vi "Process_data.vi"(4 "Measurement top level?":bool) -> (6 "Vel stat display":string[][](table), 7 "First Plot data Cluster":cluster{"X array":dbl[], "Y array":dbl[]}[](array[cluster]), 8 "Second Plot Data Cluster":cluster{"X array":dbl[], "Y array":dbl[]}[](array[cluster]), 9 "Max Measurement time up":bool)   [LabVIEW 2017]
uses:
  Controls/Instrument_Array.ctl
  Controls/Inst_type.ctl
  Controls/Post_Process.ctl
  Controls/User_Specific_mode.ctl
  Controls/Server_Comms.ctl
  Globals/Meas_global.vi
  Globals/LDA_meas_global_1.vi
  Globals/Dynamic_call_global.ph.vi
  Acquisition/PWA/PWAtasksGLOBAL.vi
  Globals/Trav_pos_global.vi
  Globals/Preference_global.vi
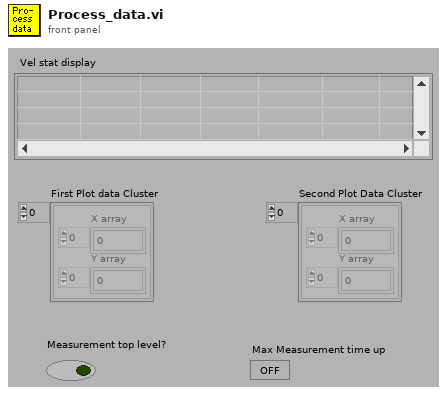
[diagram p1: front panel]
types:
  T1 = typedef "LDA_Setup.ctl" = cluster{"dimensions":enum16{"1D", "2D"}, "Analogue Freq Multiplier":dbl}
  T2 = typedef "PWA_Data.ctl" = enum16{"No PWA Data", "One Ch PWA"}
  T3 = typedef "Instrument_Array.ctl" = enum16{"PWA", "LDA", "Analogue"}
  T4 = typedef "Inst_type.ctl" = enum16{"Propeller anemometer", "Raw voltage", "Pressure Transducer", "Pitot-static tube", "Preston tube", "Hot wire", "Cross wire 1", "Cross wire 2", "Generic Linear", "Generic Polynomial", "Generic BackPoly", "Fast FID", "Thermocouple", "Cold wire", "Pulsed Wire", "LDA Vel", "LDA Tran time", "LDA Arr time", "Microphone"}
  T5 = typedef "Post_Process.ctl" = enum16{"Take New Data", "Post Process Raw Data File"}
  T6 = typedef "User_Specific_mode.ctl" = enum16{"Check VI only", "Run VI"}
  T7 = enum16{"Save no data", "Save data in new files", "Save data in existing files"}
  T8 = typedef "Server_Comms.ctl" = enum16{"Server Link Healthy", "Do Not Link To Server"}
  T9 = typedef "Trigger_Mode.ctl" = enum16{"Free Running", "Start on Trigger", "Trigger Every Block", "Trigger Every Sample"}
  T10 = typedef "Analysis_info_cluster.ctl" = cluster{"Colour":u32, "Inst type":T4, "Inst name":string, "Symbol":string, "Code name":string, "Extra Info":string, "Inst Array":T3, "Extra Titles":string[], "Extra Values":string[], "U":dbl, "u^2":dbl, "u^3":dbl, "u^4":dbl, "Skew_u":dbl, "Kurt_u":dbl, "Sd Error in Mean":dbl, "% u'/U":dbl, "X":dbl, "Y":dbl, "Z":dbl, "Timescale integral Estimate":dbl, "Sd Error in Variance":dbl, "Calib File":path, "Calib Constants":dbl[], "Output Position":bool, "Full Stats":bool, "Av Sampling Rate":dbl, "Av No of Samples":dbl, "Total Meas Time (s)":dbl, "ADAM Ch Name":string, "Max value":dbl, "Min value":dbl}
  T11 = typedef "Time_Trace_Cluster.ctl" = cluster{"Weighting":dbl[], "Time (s)":dbl[], "Voltage":dbl[], "Eng Values":dbl[]}
  T12 = typedef "Shift_Cluster.ctl" = cluster{"Stats":dbl[], "Spectra_Auto":dbl[], "Histogram":dbl[], "Hist Max":dbl, "Hist Min":dbl, "No of Samples":i32, "No in plume":i32, "Weight sum":dbl, "No Of Hist bins":i32, "TimeTrace Max":dbl, "Time Trace Min":dbl, "Trace St Deviation":dbl}
  T13 = typedef "Cross_Moments_Shift_Cluster.ctl" = cluster{"Stats":dbl[], "Resampled No of Samples":i32, "Resampled delta T":dbl, "Cross Correlation":dbl[]}
  T14 = typedef "Correlation_cluster1.ctl" = cluster{"U inst":string, "uw":dbl, "u^2w":dbl, "uw^2":dbl, "uw/u'w'":dbl, "W inst":string, "uw^3":dbl, "u^3w":dbl, "u^2w^2":dbl, "Index U":i32, "Index W":i32, "Error info":string[]}
  T15 = typedef "Traverse_cluster.ctl" = cluster{"Start X":sgl, "Start Y":sgl, "Start Z":sgl, "End X":sgl, "End Y":sgl, "End Z":sgl, "No. of pts.":i32, "Spacing":T16, "Filename":path, "Tunnel Speed":dbl, "Averaging time (min)":dbl, "Extra Commands":string, "Carrier_1 Q (l/min)":dbl, "Carrier_2 Q (l/min)":dbl, "Trace Gas Concentration (%)":dbl, "Specific Arguments":string, "Comments":string, "Row No":i32, "Row Type Selector":T17, "Completion time":string, "Row Duration (mins)":dbl, "No. of Valid pts.":i32, "Meas Setup File":string}
  T16 = typedef "Spacing.ctl" = enum16{"Linear", "Log", "Gauss", "Specified", "N/A"}
  T17 = typedef "Multi_run_mode.ctl" = enum16{"Move Traverse Only", "Set Tunnel Speed Only", "Set Source Only", "Set Measurement Conditions", "Single Measurement", "Vertical Profile", "Lateral Profile", "Longitudinal Profile", "Explore Volume", "Multi-Axis Profile", "Auto Calibrate", "Meas Fast FID Bkgnd", "Check Beam Power", "Scanning Valve Measurement", "Run VI Named:", "Set ADAM Ch", "Wait (minutes)", "Send Message", "Synchronize With:", "Fall Back to this Row", "Turn Off Row Repeating", "Blank Row", "Traverse 3D Volume"}
  T18 = typedef "Graph_Type.ctl" = enum16{"Show no graph", "Voltage trace", "Velocity trace", "Vel histogram", "Spectrum", "f.E(f) v Log f", "Auto-Corr"}
  T19 = cluster{"Plot 1":u16, "Plot 2":u16, "Save graph":u16, "Plot Type":T18}
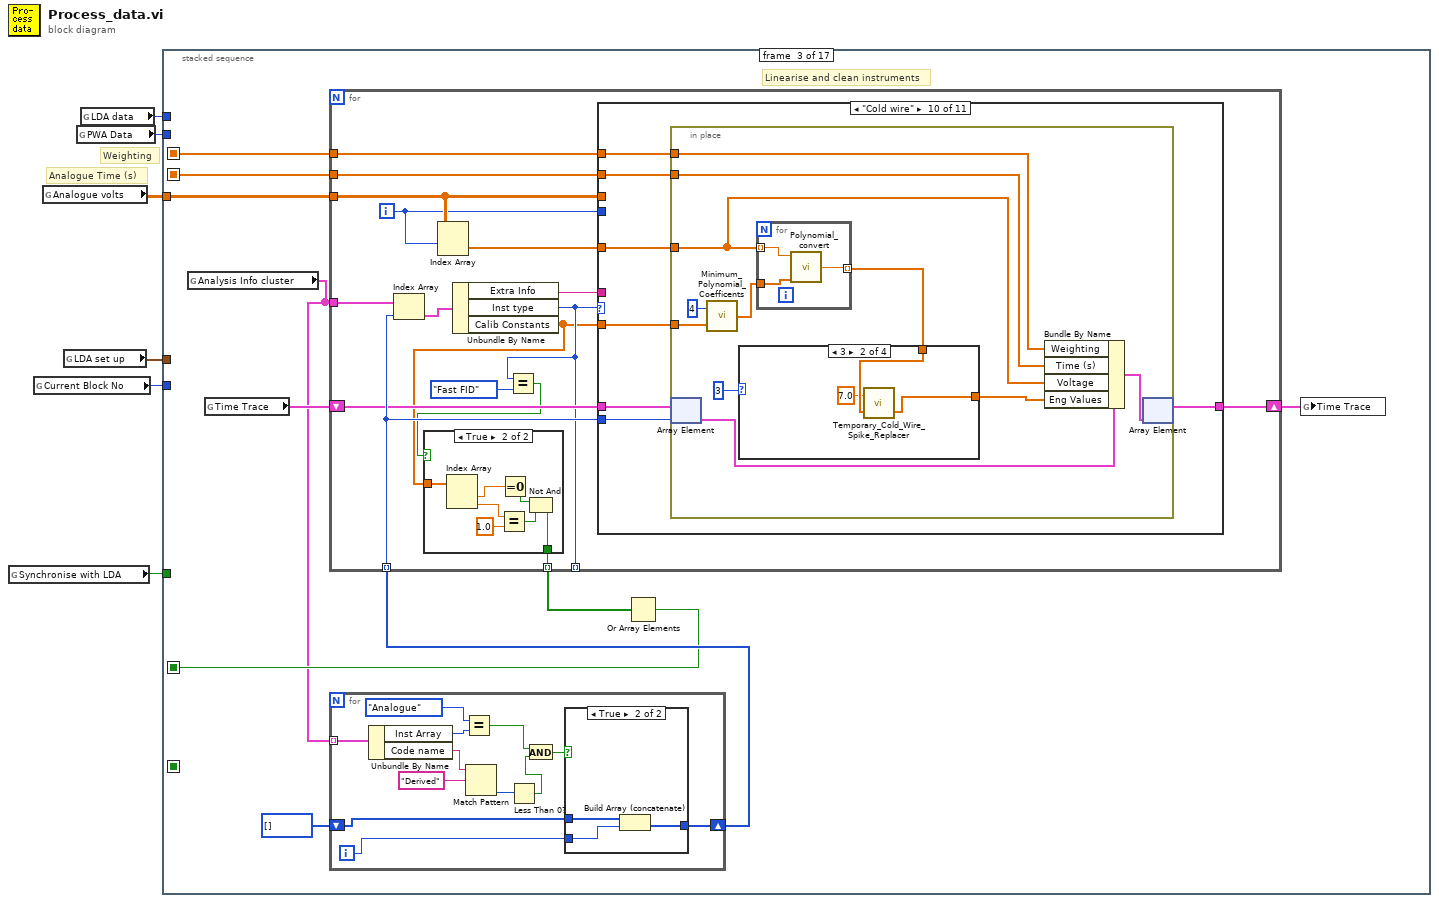
[diagram p0: block diagram]
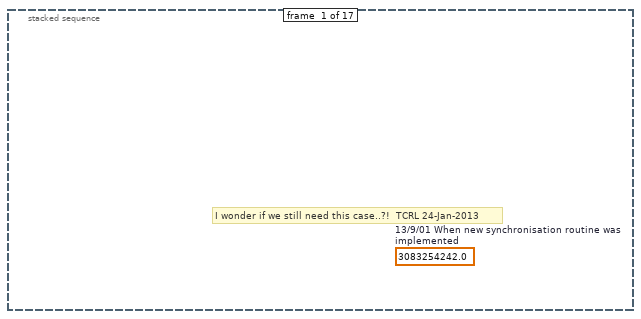
[diagram p2: hidden frame]
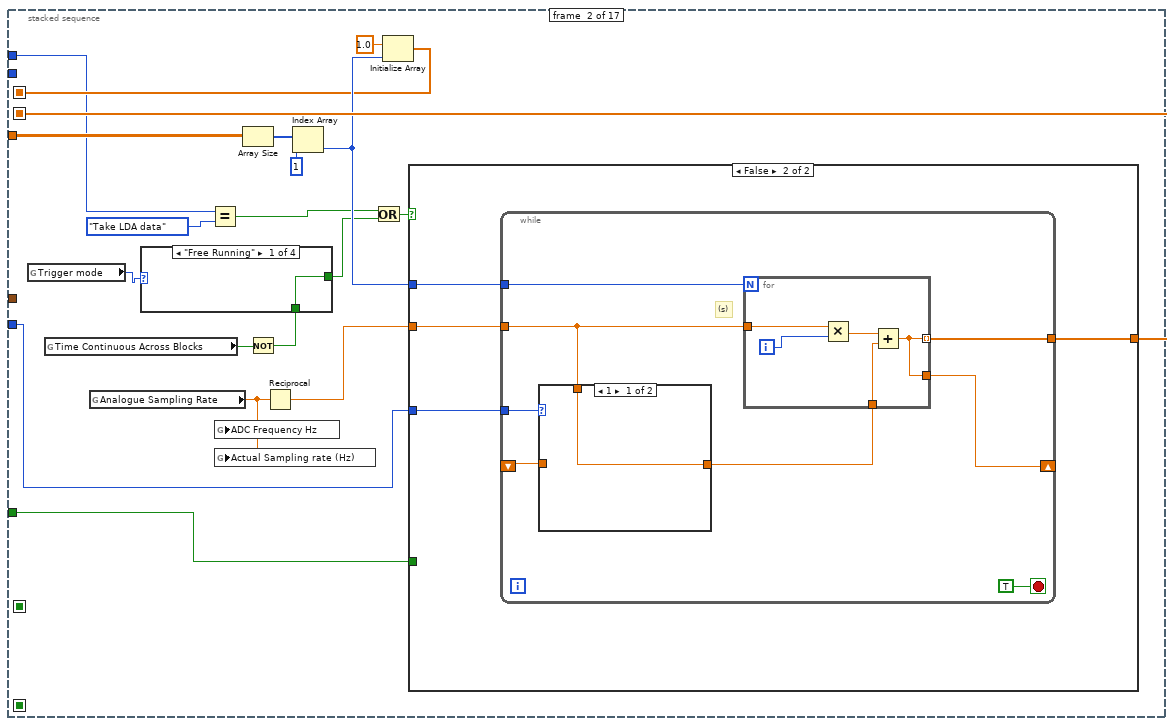
[diagram p3: hidden frame]
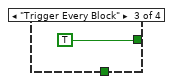
[diagram p5: hidden frame]
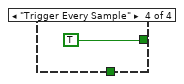
[diagram p6: hidden frame]
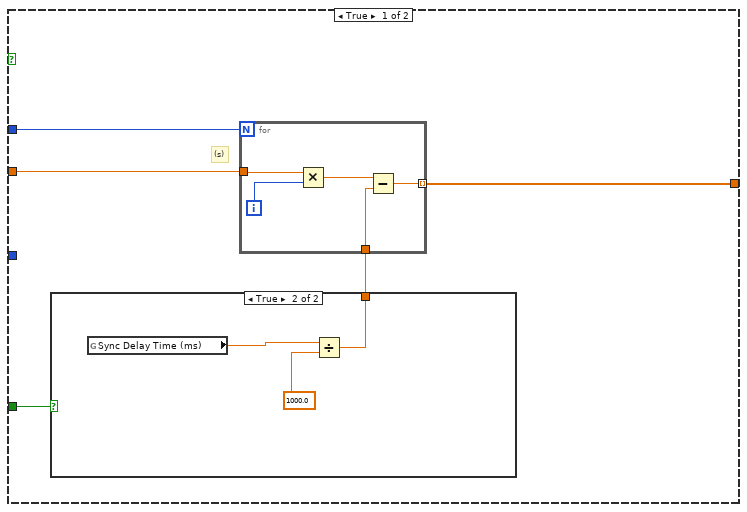
[diagram p7: hidden frame]
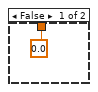
[diagram p8: hidden frame]
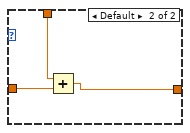
[diagram p9: hidden frame]
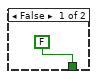
[diagram p11: hidden frame]
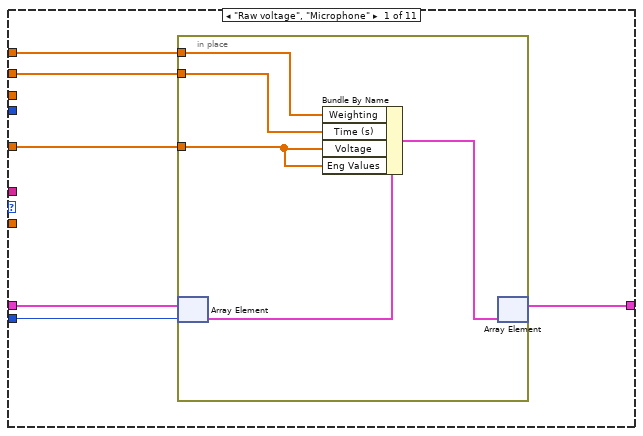
[diagram p12: hidden frame]
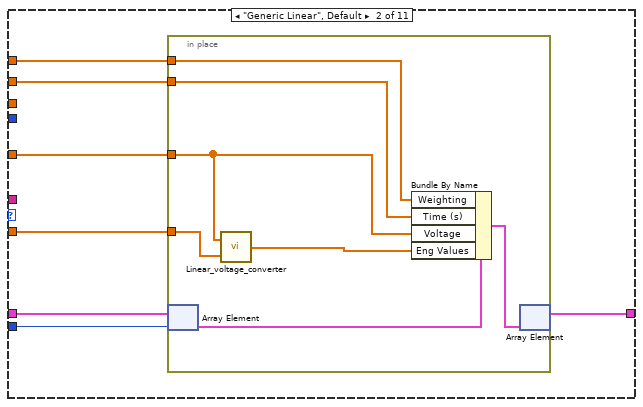
[diagram p13: hidden frame]
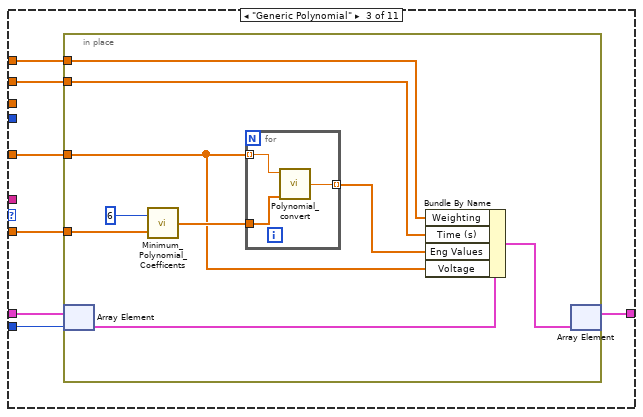
[diagram p14: hidden frame]
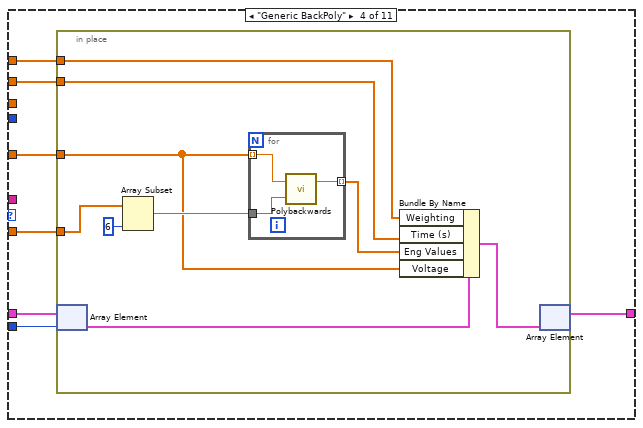
[diagram p15: hidden frame]
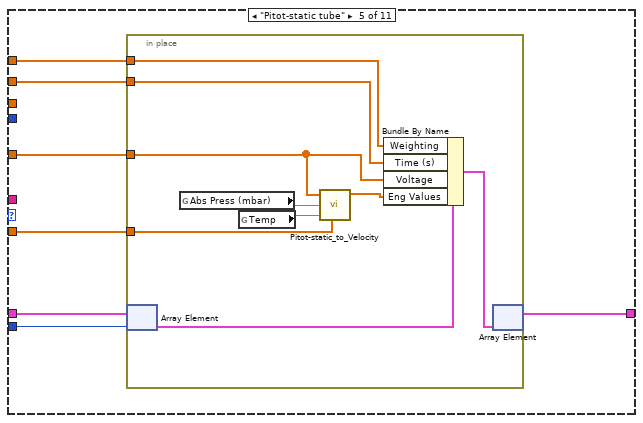
[diagram p16: hidden frame]
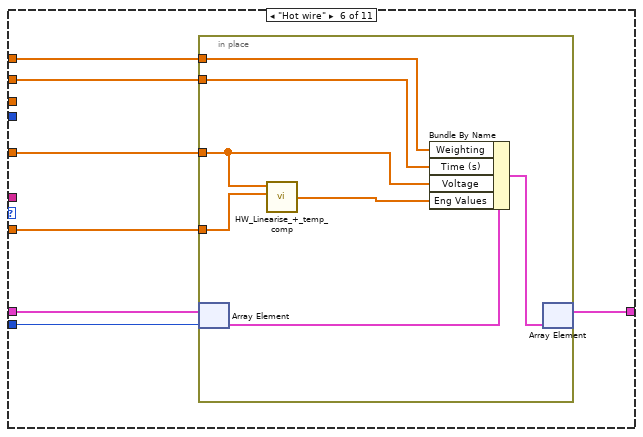
[diagram p17: hidden frame]
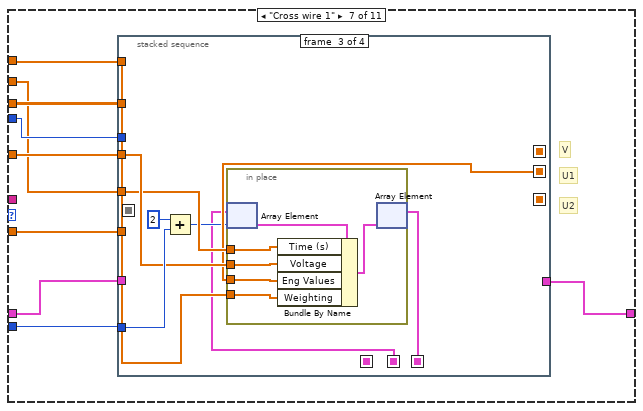
[diagram p18: hidden frame]
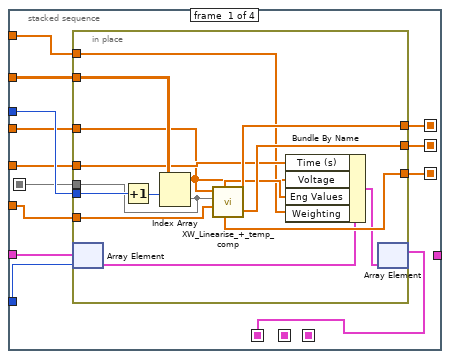
[diagram p19: hidden frame]
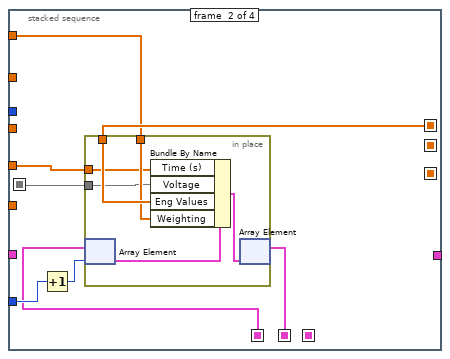
[diagram p20: hidden frame]
diagram:
  # "Weighting"
  # "Analogue Time (s)"
  n1 = global read "Meas_global.vi" "Synchronise with LDA"() -> (w4:bool)
  n2 = global read "Meas_global.vi" "Current Block No"() -> (w5:i32)
  n3 = global read "Meas_global.vi" "Analogue volts"() -> (w2:dbl[][])
  n4 = global read "Meas_global.vi" "LDA set up"() -> (w1:T1)
  n5 = global read "Meas_global.vi" "PWA Data"() -> (w3:T2)
  n6 = global read "Meas_global.vi" "LDA data"() -> (w6:enum16{"No LDA data", "Take LDA data"})
  n7 = stacked-sequence {
    seq-local: [_ w22 _ _ _ _ _ _ _ _ _ _ _ _ _ _ _] -> [_ _ w71 _ _ _ _ _ _ _ _ _ _ _ _ _ _]
    seq-local: [_ w19 _ _ _ _ _ _ _ _ _ _ _ _ _ _ _] -> [_ _ w70 _ _ _ _ _ _ _ _ _ _ _ _ _ _]
    seq-local: [_ _ w67 _ _ _ _ _ _ _ _ _ _ _ _ _ _] -> [_ _ _ _ _ w441 _ _ _ _ _ _ _ _ _ _ _]
    seq-local: [_ _ _ _ _ _ _ _ _ _ _ _ _ _ _ w709 _] -> [_ _ _ _ _ _ _ _ _ _ _ _ _ _ _ _ w735]
    tunnel: w5 -> [_ w15 _ _ _ _ w445 _ _ _ _ _ _ _ _ _ _]
    tunnel: w6 -> [_ w12 _ w383 _ _ _ _ _ _ _ _ _ _ _ w710 _]
    tunnel: w2 -> [_ w25 w74 _ _ _ _ _ _ _ _ _ w660 _ _ _ _]
    tunnel: w4 -> [_ w16 _ w382 _ _ _ _ _ _ _ _ _ _ _ _ _]
    tunnel: w3 -> [_ _ _ _ _ _ w448 _ _ _ _ _ _ _ _ _ _]
    tunnel: w1 -> [_ _ _ w380 _ _ _ _ _ _ _ _ _ _ _ _ _]
    frame #0 {
      (unwired) 3083254242.0  # 13/9/01 When new synchronisation routine was implemented
      # "I wonder if we still need this case..?!  TCRL 24-Jan-2013"
    }
    frame #1 {
      n8 = global read "Meas_global.vi" "Trigger mode"() -> (w14:T9)
      n9 = global read "Meas_global.vi" "Time Continuous Across Blocks"() -> (w8:bool)
      n10 = global read "Meas_global.vi" "Analogue Sampling Rate"() -> (w18:dbl)
      n11 = Equal?(x=w12, y=enum16{"No LDA data", "Take LDA data"}."Take LDA data" ("LDA data")) -> (x = y?=w10:bool)
      n12 = global write "LDA_meas_global_1.vi" "ADC Frequency Hz"(w18) -> ()
      n13 = global write "Meas_global.vi" "Actual Sampling rate (Hz)"(w18) -> ()
      n14 = Array Size(array=w25) -> (size(s)=w24:i32[])
      n15 = Not(x=w8) -> (.not. x?=w7:bool)
      n16 = case shown="\"Free Running\"" w14 {
        tunnel: [w26 w27 TRUE TRUE] -> w9
        tunnel: w7 -> [w26 w27 _ _]
        frame "Free Running" {
        }
        frame "Start on Trigger" {
        }
        frame "Trigger Every Block" {
        }
        frame "Trigger Every Sample" {
        }
      }
      n17 = Reciprocal(x=w18) -> (1/x=w17:dbl)
      n18 = Index Array(array=w24, index=1) -> (element=w21:i32)
      n19 = Or(x=w10, y=w9) -> (x .or. y?=w11:bool)
      n20 = Initialize Array(1.0 ("element"), w21) -> (w19:dbl[])
      n21 = case shown="False" w11 {
        tunnel: [w34 w47] -> w22
        tunnel: w21 -> [w33 w46]
        tunnel: w17 -> [w31 w45]
        tunnel: w16 -> [w30 _]
        tunnel: w15 -> [_ w44]
        frame True {
          # "(s)"
          n22 = case shown="True" w30 {
            tunnel: [0.0 w37] -> w32
            frame False {
            }
            frame True {
              n23 = global read "LDA_meas_global_1.vi" "Sync Delay Time (ms)"() -> (w38:dbl)
              n24 = Divide(x=w38, y=1000.0) -> (x/y=w37:dbl)
            }
          }
          n25 = for {
            N: w33 -> [_]
            tunnel: w31 -> [w42]
            tunnel: [w41] -> w34 mode=indexing
            tunnel: w32 -> [w39]
            i -> [w43]
            n26 = Multiply(x=w42, y=w43) -> (x*y=w40:dbl)
            n27 = Subtract(x=w40, y=w39) -> (x-y=w41:dbl)
          }
        }
        frame False {
          n28 = while {
            tunnel: [w55] -> w47
            tunnel: w46 -> [w54]
            tunnel: w45 -> [w48]
            tunnel: w44 -> [w52]
            shift-right: [w50] -> _
            shift-left: _ -> [w49]
            stop <- TRUE stop-if-true
            # "(s)"
            n29 = case shown="1" w52 {
              tunnel: [w56 w57] -> w51
              tunnel: w49 -> [_ w59]
              tunnel: w48 -> [w56 w58]
              frame 1 {
              }
              frame Default {
                n30 = Add(x=w58, y=w59) -> (x+y=w57:dbl)
              }
            }
            n31 = for {
              N: w54 -> [_]
              tunnel: w48 -> [w64]
              tunnel: [w61] -> w55 mode=indexing
              tunnel: w51 -> [w62]
              tunnel: [w61] -> w50
              i -> [w60]
              n32 = Multiply(x=w64, y=w60) -> (x*y=w63:dbl)
              n33 = Add(x=w63, y=w62) -> (x+y=w61:dbl)
            }
          }
        }
      }
    }
    frame #2 {
      # "Linearise and clean instruments"
      n34 = global read "Meas_global.vi" "Analysis Info cluster"() -> (w66:T10[])
      n35 = global read "Meas_global.vi" "Time Trace"() -> (w69:T11[])
      n36 = for {
        tunnel: w66 -> [w78] mode=indexing
        shift-right: [w75] -> w72
        shift-left: i32[] [] -> [w76]
        i -> [w77]
        n37 = Unbundle By Name(w78) -> ("Inst Array"=w86:T3, "Code name"=w84:string)
        n38 = Equal?(x=Instrument_Array."Analogue" ("Inst Array"), y=w86) -> (x = y?=w80:bool)
        n39 = Match Pattern(string=w84, regular expression="Derived") -> (offset past match=w82:i32)  [unwired: 4 out]
        n40 = Less Than 0?(x=w82) -> (x < 0?=w81:bool)
        n41 = And(x=w80, y=w81) -> (x .and. y?=w79:bool)
        n42 = case shown="True" w79 {
          tunnel: w77 -> [_ w90]
          tunnel: w76 -> [w87 w89]
          tunnel: [w87 w88] -> w75
          frame False {
          }
          frame True {
            n43 = Build Array (concatenate)(w89, w90) -> (w88:i32[])
          }
        }
      }
      n44 = for {
        tunnel: w74 -> [w106]
        tunnel: [w94] -> _ mode=indexing
        tunnel: w72 -> [w102] mode=indexing
        shift-right: [w98] -> w68
        shift-left: w69 -> [w101]
        tunnel: w71 -> [w99]
        tunnel: w70 -> [w105]
        tunnel: w66 -> [w104]
        tunnel: [w91] -> w65 mode=indexing
        i -> [w97]
        n45 = Index Array(array=w104, index=w102) -> (element=w103:T10)
        n46 = Index Array(array=w106, index (row)=w97) -> (element=w100:dbl[])  [unwired: 1 in]
        n47 = Unbundle By Name(w103) -> ("Extra Info"=w96:string, "Inst type"=w94:T4, "Calib Constants"=w93:dbl[])
        n48 = Equal?(x=w94, y=Inst_type."Fast FID" ("Inst type")) -> (x = y?=w92:bool)
        n49 = case shown="True" w92 {
          tunnel: w93 -> [_ w114]
          tunnel: [FALSE w108] -> w91
          frame False {
          }
          frame True {
            n50 = Index Array(array=w114) -> (element #1=w113:dbl, element #2=w112:dbl)  [unwired: 2 in]
            n51 = Equal?(x=w112, y=1.0) -> (x = y?=w110:bool)
            n52 = Equal To 0?(x=w113) -> (x = 0?=w109:bool)
            n53 = Not And(1:w110, 2:w109) -> (0:w108:bool)
          }
        }
        n54 = case shown="\"Cold wire\"" w94 {
          tunnel: w93 -> [_ w132 w145 w165 w184 w200 w215 _ w295 w326 w363]
          tunnel: w97 -> [_ _ _ _ _ _ w216 _ _ _ _]
          tunnel: w106 -> [_ _ _ _ _ _ w213 _ _ _ _]
          tunnel: w99 -> [w115 w126 w144 w161 w178 w194 w210 _ w290 w322 w357]
          tunnel: w100 -> [w116 w131 w146 w164 w183 w199 w214 _ w294 w327 w362]
          tunnel: w102 -> [w119 w130 w142 w162 w180 w195 w212 _ w292 w321 w359]
          tunnel: w101 -> [w120 w128 w141 w163 w181 w197 w211 w288 w293 w325 w360]
          tunnel: [w117 w127 w140 w159 w179 w196 w209 w288 w291 w324 w358] -> w98
          tunnel: w105 -> [w118 w129 w143 w160 w182 w198 w208 _ w289 w323 w361]
          tunnel: w96 -> [_ _ _ _ _ _ _ _ _ _ w356]
          frame "Raw voltage", "Microphone" {
            n55 = in-place {
              in-place-border: w118 -> [w121]
              in-place-border: w116 -> [w123]
              in-place-border: w115 -> [w122]
              n56 = in-place-array #1(w120, w119) -> (w124:T11)
              n57 = Bundle By Name(cluster=w124, "Weighting"=w121, "Time (s)"=w122, "Voltage"=w123, "Eng Values"=w123) -> (w125:T11)
              n58 = in-place-array #1(w125) -> (w117:T11[])  [unwired: 1 out]
            }
          }
          frame "Generic Linear", Default {
            n59 = in-place {
              in-place-border: w132 -> [w139]
              in-place-border: w131 -> [w134]
              in-place-border: w129 -> [w133]
              in-place-border: w126 -> [w135]
              n60 = in-place-array #2(w128, w130) -> (w136:T11)
              n61 = call "Linear_voltage_converter.vi"("Caib const A,B"=w139, "Voltage array"=w134) -> ("Converted array"=w138:dbl[])
              n62 = Bundle By Name(cluster=w136, "Weighting"=w133, "Time (s)"=w135, "Voltage"=w134, "Eng Values"=w138) -> (w137:T11)
              n63 = in-place-array #2(w137) -> (w127:T11[])  [unwired: 1 out]
            }
          }
          frame "Generic Polynomial" {
            n64 = in-place {
              in-place-border: w146 -> [w151]
              in-place-border: w145 -> [w154]
              in-place-border: w144 -> [w148]
              in-place-border: w143 -> [w147]
              n65 = in-place-array #3(w141, w142) -> (w150:T11)
              n66 = call "Minimum_Polynomial_Coefficents.vi"("Calib consts"=w154, "Max Length"=6) -> ("Coefficients"=w153:dbl[])
              n67 = for {
                tunnel: w153 -> [w158]
                tunnel: w151 -> [w157] mode=indexing
                tunnel: [w156] -> w152 mode=indexing
                n68 = call "Polynomial_convert.vi"("Calib constants"=w158, "Voltage"=w157) -> ("Eng Values"=w156:dbl)  [unwired: 4 out]
              }
              n69 = Bundle By Name(cluster=w150, "Weighting"=w147, "Time (s)"=w148, "Eng Values"=w152, "Voltage"=w151) -> (w149:T11)
              n70 = in-place-array #3(w149) -> (w140:T11[])  [unwired: 1 out]
            }
          }
          frame "Generic BackPoly" {
            n71 = in-place {
              in-place-border: w165 -> [w174]
              in-place-border: w164 -> [w169]
              in-place-border: w161 -> [w167]
              in-place-border: w160 -> [w166]
              n72 = in-place-array #4(w163, w162) -> (w171:T11)
              n73 = Array Subset(array=w174, length=6) -> (w173:dbl[])  [unwired: 1 in]
              n74 = for {
                tunnel: w173 -> [w177]
                tunnel: w169 -> [w176] mode=indexing
                tunnel: [w175] -> w170 mode=indexing
                n75 = call "Polybackwards.vi"("Coefficients"=w177, "Y input"=w176) -> ("X output"=w175:dbl)  [unwired: 1 out]
              }
              n76 = Bundle By Name(cluster=w171, "Weighting"=w166, "Time (s)"=w167, "Eng Values"=w170, "Voltage"=w169) -> (w168:T11)
              n77 = in-place-array #4(w168) -> (w159:T11[])  [unwired: 1 out]
            }
          }
          frame "Pitot-static tube" {
            n78 = in-place {
              in-place-border: w184 -> [w193]
              in-place-border: w183 -> [w187]
              in-place-border: w182 -> [w185]
              in-place-border: w178 -> [w188]
              n79 = in-place-array #5(w181, w180) -> (w190:T11)
              n80 = global read "Meas_global.vi" "Abs Press (mbar)"() -> (w192:dbl)
              n81 = global read "Meas_global.vi" "Temp"() -> (w186:dbl)
              n82 = call "Pitot-static_to_Velocity.vi"("Pressure Trans voltage"=w187, "Atmos Press mbar  (1000)"=w192, "Temp  C  (20)"=w186, "Pressure Trans Calib const"=w193) -> ("Velocity (m/s)"=w191:dbl[])  [unwired: 1 in, 3 out]
              n83 = Bundle By Name(cluster=w190, "Weighting"=w185, "Time (s)"=w188, "Voltage"=w187, "Eng Values"=w191) -> (w189:T11)
              n84 = in-place-array #5(w189) -> (w179:T11[])  [unwired: 1 out]
            }
          }
          frame "Hot wire" {
            n85 = in-place {
              in-place-border: w200 -> [w207]
              in-place-border: w199 -> [w202]
              in-place-border: w198 -> [w201]
              in-place-border: w194 -> [w203]
              n86 = in-place-array #6(w197, w195) -> (w205:T11)
              n87 = call "HW_Linearise_+_temp_comp.vi"("Caib const"=w207, "HW voltage"=w202) -> ("Velocity"=w206:dbl[])  [unwired: 3 in, 1 out]
              n88 = Bundle By Name(cluster=w205, "Weighting"=w201, "Time (s)"=w203, "Voltage"=w202, "Eng Values"=w206) -> (w204:T11)
              n89 = in-place-array #6(w204) -> (w196:T11[])  [unwired: 1 out]
            }
          }
          frame "Cross wire 1" {
            # "U2"
            # "U1"
            # "V"
            n90 = stacked-sequence {
              seq-local: [w225 _ _ _] -> [_ w250 _ _]
              seq-local: [w224 _ _ _] -> [_ _ w262 _]
              seq-local: [w223 _ _ _] -> [_ _ _ w278]
              seq-local: [_ w245 _ _] -> [_ _ w259 _]
              seq-local: [_ _ w258 _] -> [_ _ _ w274]
              seq-local: [w222 _ _ _] -> [_ w248 _ w277]
              seq-local: [w219 _ _ _] -> [_ w244 _ _]
              tunnel: w216 -> [w229 _ _ _]
              tunnel: w215 -> [w228 _ _ _]
              tunnel: w214 -> [w227 _ w265 _]
              tunnel: w213 -> [w226 _ _ _]
              tunnel: w212 -> [w220 w251 w266 w281]
              tunnel: w211 -> [w221 _ _ _]
              tunnel: w210 -> [w218 w247 w264 w280]
              tunnel: [_ _ _ w273] -> w209
              tunnel: w208 -> [w217 w249 w261 w276]
              frame #0 {
                n91 = in-place {
                  in-place-border: w229 -> [w243]
                  in-place-border: w228 -> [w241]
                  in-place-border: w227 -> [w230]
                  in-place-border: w226 -> [w240]
                  in-place-border: [w239] -> w225
                  in-place-border: [w238] -> w224
                  in-place-border: [w237] -> w223
                  in-place-border: [w236] -> w222
                  in-place-border: w218 -> [w232]
                  in-place-border: w217 -> [w231]
                  n92 = in-place-array #7(w221, w220) -> (w233:T11)
                  n93 = Increment(x=w243) -> (x+1=w242:i32)
                  n94 = Index Array(array=w240, index (row)=w242) -> (element=w236:dbl[])  [unwired: 1 in]
                  n95 = call "XW_Linearise_+_temp_comp.vi"("Calib const"=w241, "XW2 voltage"=w236, "XW1 voltage"=w230) -> ("U1"=w238:dbl[], "V"=w239:dbl[], "U2"=w237:dbl[], "U"=w235:dbl[])  [unwired: 1 in]
                  n96 = Bundle By Name(cluster=w233, "Time (s)"=w232, "Voltage"=w230, "Eng Values"=w235, "Weighting"=w231) -> (w234:T11)
                  n97 = in-place-array #7(w234) -> (w219:T11[])  [unwired: 1 out]
                }
              }
              frame #1 {
                n98 = Increment(x=w251) -> (x+1=w246:i32)
                n99 = in-place {
                  in-place-border: w250 -> [w257]
                  in-place-border: w249 -> [w256]
                  in-place-border: w248 -> [w255]
                  in-place-border: w247 -> [w254]
                  n100 = in-place-array #8(w244, w246) -> (w253:T11)
                  n101 = Bundle By Name(cluster=w253, "Time (s)"=w254, "Voltage"=w255, "Eng Values"=w257, "Weighting"=w256) -> (w252:T11)
                  n102 = in-place-array #8(w252) -> (w245:T11[])  [unwired: 1 out]
                }
              }
              frame #2 {
                n103 = Add(x=2, y=w266) -> (x+y=w260:i32)
                n104 = in-place {
                  in-place-border: w265 -> [w272]
                  in-place-border: w264 -> [w271]
                  in-place-border: w262 -> [w270]
                  in-place-border: w261 -> [w269]
                  n105 = in-place-array #9(w259, w260) -> (w268:T11)
                  n106 = Bundle By Name(cluster=w268, "Time (s)"=w271, "Voltage"=w272, "Eng Values"=w270, "Weighting"=w269) -> (w267:T11)
                  n107 = in-place-array #9(w267) -> (w258:T11[])  [unwired: 1 out]
                }
              }
              frame #3 {
                n108 = Add(x=3, y=w281) -> (x+y=w275:i32)
                n109 = in-place {
                  in-place-border: w280 -> [w287]
                  in-place-border: w278 -> [w286]
                  in-place-border: w277 -> [w285]
                  in-place-border: w276 -> [w284]
                  n110 = in-place-array #10(w274, w275) -> (w283:T11)
                  n111 = Bundle By Name(cluster=w283, "Time (s)"=w287, "Voltage"=w285, "Eng Values"=w286, "Weighting"=w284) -> (w282:T11)
                  n112 = in-place-array #10(w282) -> (w273:T11[])  [unwired: 1 out]
                }
              }
            }
          }
          frame "Cross wire 2" {
          }
          frame "Fast FID" {
            n113 = in-place {
              in-place-border: w295 -> [w307]
              in-place-border: w294 -> [w298]
              in-place-border: w292 -> [w302]
              in-place-border: w290 -> [w297]
              in-place-border: w289 -> [w296]
              n114 = in-place-array #11(w293, w292) -> (w300:T11)
              n115 = global read "LDA_meas_global_1.vi" "ADC Frequency Hz"() -> (w303:dbl)
              n116 = Array Subset(array=w307, length=3) -> (w306:dbl[])  [unwired: 1 in]
              n117 = call "2nd_order_Poly_convert.vi"("Calib constants"=w306, "Voltage"=w298) -> ("Eng Values"=w305:dbl[])  [unwired: 4 out]
              n118 = Index Array(array=w307, index=3) -> (element=w313:dbl)
              n119 = Index Array(array=w307, index=4) -> (element=w309:dbl)
              n120 = Subtract(x=w305, y=w313) -> (x-y=w312:dbl[])
              n121 = Greater?(x=w303, y=90.0) -> (0:w304:bool)
              n122 = case shown="True" w304 {
                tunnel: w312 -> [w315 w320]
                tunnel: [w315 w319] -> w301
                tunnel: w309 -> [_ w318]
                tunnel: w303 -> [_ w317]
                tunnel: w302 -> [_ w316]
                frame False {
                }
                frame True {
                  n123 = call "Remove_FF_lone_spikes.vi"("ADC Frequency Hz"=w317, "Bkgnd variance"=w318, "AIC index"=w316, "Time Trace"=w320) -> ("Filtered Time Trace"=w319:dbl[])  [unwired: 1 in, 1 out]
                }
              }
              n124 = Bundle By Name(cluster=w300, "Weighting"=w296, "Time (s)"=w297, "Voltage"=w298, "Eng Values"=w301) -> (w299:T11)
              n125 = in-place-array #11(w299) -> (w291:T11[])  [unwired: 1 out]
            }
          }
          frame "Cold wire" {
            n126 = in-place {
              in-place-border: w327 -> [w330]
              in-place-border: w326 -> [w337]
              in-place-border: w323 -> [w328]
              in-place-border: w322 -> [w329]
              n127 = in-place-array #12(w325, w321) -> (w331:T11)
              n128 = call "Minimum_Polynomial_Coefficents.vi"("Calib consts"=w337, "Max Length"=4) -> ("Coefficients"=w336:dbl[])
              n129 = for {
                tunnel: w336 -> [w355]
                tunnel: w330 -> [w354] mode=indexing
                tunnel: [w353] -> w335 mode=indexing
                n130 = call "Polynomial_convert.vi"("Calib constants"=w355, "Voltage"=w354) -> ("Eng Values"=w353:dbl)  [unwired: 4 out]
              }
              n131 = case shown="3" 3 {
                tunnel: w335 -> [w339 w342 w345 w350]
                tunnel: [w339 w341 w343 w349] -> w333
                frame 0, Default {
                }
                frame 3 {
                  n132 = call "Temporary_Cold_Wire_Spike_Replacer.vi"("Data in"=w342, "St Dev threshold"=7.0) -> ("Data out"=w341:dbl[])  [unwired: 1 out]
                }
                frame 1 {
                  n133 = global read "LDA_meas_global_1.vi" "ADC Frequency Hz"() -> (w346:dbl)
                  n134 = Reciprocal(x=w346) -> (1/x=w347:dbl)
                  n135 = call "Ideal_LowPass_Filter_PN.vi"("Cutoff frequency (Hz)"=100.0, "dt (s)"=w347, "1D Data (uniform spacing)"=w345) -> ("Low-pass filtered 1D Data"=w343:dbl[])
                }
                frame 2 {
                  n136 = global read "LDA_meas_global_1.vi" "ADC Frequency Hz"() -> (w351:dbl)
                  n137 = Reciprocal(x=w351) -> (1/x=w352:dbl)
                  n138 = call "Ideal_Notch_Filter_PN.vi"("Frequencies to cut (Hz)"=dbl[] [150.0, 250.0], "dt (s)"=w352, "1D Data (uniform spacing)"=w350) -> ("Low-pass filtered 1D Data"=w349:dbl[])
                }
              }
              n139 = Bundle By Name(cluster=w331, "Weighting"=w328, "Time (s)"=w329, "Voltage"=w330, "Eng Values"=w333) -> (w332:T11)
              n140 = in-place-array #12(w332) -> (w324:T11[])  [unwired: 1 out]
            }
          }
          frame "Preston tube" {
            n141 = in-place {
              in-place-border: w363 -> [w379]
              in-place-border: w362 -> [w366]
              in-place-border: w361 -> [w364]
              in-place-border: w357 -> [w367]
              in-place-border: w356 -> [w365]
              w375 = 0.0  # Static gauge press mm H2O
              n142 = in-place-array #13(w360, w359) -> (w369:T11)
              n143 = global read "Meas_global.vi" "Abs Press (mbar)"() -> (w378:dbl)
              n144 = global read "Meas_global.vi" "Temp"() -> (w372:dbl)
              n145 = Match Pattern(string=w365, regular expression="D = " ("String to match")) -> (after substring=w376:string)  [unwired: 4 out]
              n146 = call "String_2_Number.vi"("Value"=w376) -> ("Numeric"=w371:dbl)
              n147 = Array Size(array=w366) -> (size(s)=w374:i32)
              n148 = call "Preston_shear_stress.vi"("Calib. consts"=w379, "Diam. (mm)"=w371, "Temp (C)"=w372, "Static gauge head mm H2O"=w375, "Atmos. pressure (mbars)"=w378, "Pressure transducer voltages"=w366) -> ("Mean shear stress (Pa)"=w373:dbl)  [unwired: 1 in, 3 out]
              n149 = Initialize Array(w373, w374) -> (w370:dbl[])
              n150 = Bundle By Name(cluster=w369, "Weighting"=w364, "Time (s)"=w367, "Voltage"=w366, "Eng Values"=w370) -> (w368:T11)
              n151 = in-place-array #13(w368) -> (w358:T11[])  [unwired: 1 out]
            }
          }
        }
      }
      n152 = Or Array Elements(Boolean array=w65) -> (logical OR=w67:bool)
      n153 = global write "Meas_global.vi" "Time Trace"(w68) -> ()
    }
    frame #3 {
      n154 = Unbundle By Name(w380) -> ("dimensions"=w381:enum16{"1D", "2D"})
      n155 = case shown="\"Take LDA data\"" w383 {
        tunnel: w381 -> [_ w385]
        tunnel: w382 -> [_ w384]
        frame "No LDA data" {
        }
        frame "Take LDA data" {
          # "New Sync"
          n156 = stacked-sequence {
            seq-local: [w389 _ _] -> [_ w392 w394]
            tunnel: w385 -> [_ w393 _]
            tunnel: w384 -> [w390 _ _]
            frame #0 {
              w387 = 3083254242.0  # 13/9/01 When new synchronisation routine was implemented
              n157 = global read "Meas_global.vi" "Time Data was Aquired"() -> (w388:dbl)
              n158 = Greater?(x=w388, y=w387) -> (0:w386:bool)
              n159 = Compound Arithmetic op=AND(w390, w386) -> (w389:bool)
            }
            frame #1 {
              n160 = Not(x=w392) -> (.not. x?=w391:bool)
              n161 = call "LDA_High_Convert_New.vi"("dimensions"=w393, "Create Sync Index"=w391) -> ()  [unwired: 1 in, 4 out]
            }
            frame #2 {
              n162 = case shown="True" w394 {
                frame False {
                }
                frame True {
                  n163 = global read "Meas_global.vi" "Time Trace"() -> (w398:T11[])
                  n164 = global read "Meas_global.vi" "Analysis Info cluster"() -> (w396:T10[])
                  n165 = for {
                    tunnel: w396 -> [w426] mode=indexing
                    tunnel: [w417] -> w399
                    tunnel: w398 -> [w418] mode=indexing
                    stop <- w419 stop-if-true
                    n166 = Unbundle By Name(w418) -> ("Eng Values"=w417:dbl[])
                    n167 = Unbundle By Name(w426) -> ("Inst type"=w424:T4, "Symbol"=w422:string)  [unwired: 1 out]
                    n168 = Equal?(x=Inst_type."Raw voltage" ("Inst type"), y=w424) -> (x = y?=w420:bool)
                    n169 = Equal?(x="Sync", y=w422) -> (x = y?=w421:bool)
                    n170 = And(x=w420, y=w421) -> (x .and. y?=w419:bool)
                  }
                  n171 = global read "Meas_global.vi" "Analogue Sampling Rate"() -> (w401:dbl)
                  n172 = global read "LDA_meas_global_1.vi" "Arrival times"() -> (w400:dbl[])
                  n173 = Reciprocal(x=w401) -> (1/x=w402:dbl)
                  n174 = call "LDA_analogue_start_time_sync_PN.vi"("Analogue dt (s)"=w402, "Analogue LDA burst pulse array (s)"=w399, "LDA arrival times (s)"=w400) -> ("LDA start time rel. to Analogue (s)"=w395:dbl)  [unwired: 7 in, 1 out]
                  n175 = for {
                    tunnel: w396 -> [w407] mode=indexing
                    tunnel: w395 -> [w408]
                    tunnel: [w406] -> w397 mode=indexing
                    tunnel: w398 -> [w403] mode=indexing
                    n176 = Unbundle By Name(w407) -> ("Inst Array"=w410:T3)
                    n177 = Unbundle By Name(w403) -> ("Time (s)"=w404:dbl[])
                    n178 = Equal?(x=Instrument_Array."LDA" ("Inst Array"), y=w410) -> (x = y?=w405:bool)
                    n179 = case shown="True" w405 {
                      tunnel: w408 -> [_ w416]
                      tunnel: w404 -> [_ w415]
                      tunnel: w403 -> [w411 w414]
                      tunnel: [w411 w412] -> w406
                      frame False {
                      }
                      frame True {
                        n180 = Add(x=w416, y=w415) -> (x+y=w413:dbl[])
                        n181 = Bundle By Name(cluster=w414, "Time (s)"=w413) -> (w412:T11)
                      }
                    }
                  }
                  n182 = global write "Meas_global.vi" "Time Trace"(w397) -> ()
                }
              }
            }
          }
        }
      }
    }
    frame #4 {
      n183 = global read "Dynamic_call_global.ph.vi" "Pre_Analysis_Plugin"() -> (w428:string)
      n184 = Empty String/Path?(string/path=w428) -> (empty?=w427:bool)
      n185 = case shown="True" w427 {
        tunnel: w428 -> [w432 _]
        frame False {
          w436 = FALSE  # Dialog Box (T)
          n186 = call "Plug_in_Directories.vi"() -> ("Pre_Analysis_Plugins"=w429:path)  [unwired: 2 in, 4 out]
          n187 = Build Path(base path=w429, name or relative path=w432) -> (appended path=w434:path)
          n188 = Open VI Reference(type specifier VI Refnum (for type only)=refnum<vi> refnum ("Plug in"), vi path=w434) -> (vi reference=w440:refnum<vi>, error out=w439:errorcluster)  [unwired: 2 in, 2 out]
          n189 = call-by-ref "?"(reference=w440, error in=w439) -> (reference out=w437:refnum<vi>, error out=w438:errorcluster)  [unwired: 1 in]
          n190 = Concatenate Strings("Running Pre_Analysis Plugin named" ("Error Type"), w432) -> (w430:string)
          n191 = Close Reference(reference=w437, error in (no error)=w438) -> (error out=w435:errorcluster)
          n192 = call "EnFlo_Error_Handler.vi"("error in (no error)"=w435, "Error Type"=w430, "Dialog Box (T)"=w436) -> ()  [unwired: 3 out]
        }
        frame True {
        }
      }
    }
    frame #5 {
      n193 = case shown="True" w441 {
        frame False {
        }
        frame True {
          # "This must not run until the Time trace global has been populated"
          n194 = call "FF_Bkgnd_correction.vi"() -> ()  [unwired: 1 in, 3 out]
        }
      }
    }
    frame #6 {
      n195 = case shown="\"One Ch PWA\"" w448 {
        tunnel: [w450 w462] -> w447
        tunnel: [w450 w461] -> w446
        tunnel: w445 -> [_ w457]
        tunnel: [w449 w455] -> w443
        tunnel: [w449 w454] -> w444
        tunnel: [w449 w452] -> w442
        frame "No PWA Data" {
          w449 = 0 ("y")
          w450 = dbl[][] []
        }
        frame "One Ch PWA" {
          n196 = global read "PWAtasksGLOBAL.vi" "PWA Binary"() -> (w451:i16[][])
          n197 = global read "PWAtasksGLOBAL.vi" "Minimum TOF Index"() -> (w460:i16)
          n198 = global read "PWAtasksGLOBAL.vi" "PWA Lookup Table"() -> (w459:dbl[])
          n199 = Equal?(x=w457, y=1) -> (x = y?=w453:bool)
          n200 = Index Array(array=w451, index (row)=0) -> (element=w465:i16[])  [unwired: 1 in]
          n201 = global read "PWAtasksGLOBAL.vi" "PWA Seconds per clock pulse"() -> (w458:dbl)
          n202 = for {
            tunnel: w465 -> [w484] mode=indexing
            tunnel: [w486] -> w464 mode=indexing
            tunnel: [w485] -> w463 mode=indexing
            tunnel: w460 -> [w483]
            tunnel: w459 -> [w482]
            tunnel: w458 -> [w481]
            shift-right: [w480] -> w455
            shift-left: _ -> [w478]
            shift-right: [w479] -> w454
            shift-left: _ -> [w477]
            tunnel: w453 -> [w474]
            shift-right: [w468] -> w452
            shift-left: _ -> [w470]
            i -> [w476]
            w467 = 0 ("y")
            n203 = Equal To 0?(x=w476) -> (x = 0?=w475:bool)
            n204 = And(x=w474, y=w475) -> (x .and. y?=w471:bool)
            n205 = Select(t=w467, s=w471, f=w470) -> (s? t:f=w469:i32)
            n206 = Select(t=w467, s=w471, f=w478) -> (s? t:f=w473:i32)
            n207 = Select(t=w467, s=w471, f=w477) -> (s? t:f=w472:i32)
            n208 = case shown="0, Default" w484 {
              tunnel: w484 -> [w494 _ _]
              tunnel: [w499 w532 w537] -> w486
              tunnel: [w500 w532 w537] -> w485
              tunnel: w483 -> [w498 _ _]
              tunnel: w482 -> [w496 _ _]
              tunnel: w481 -> [w493 _ _]
              tunnel: w473 -> [w492 w531 w536]
              tunnel: [w491 w530 w535] -> w480
              tunnel: [w489 w529 w534] -> w479
              tunnel: w472 -> [w490 w529 w534]
              tunnel: w469 -> [w488 w528 w533]
              tunnel: [w487 w528 w533] -> w468
              frame 0, Default {
                n209 = Absolute Value(x=w494) -> (abs(x)=w495:i16)
                n210 = Greater?(x=w495, y=w498) -> (0:w497:bool)
                n211 = case shown="True" w497 {
                  tunnel: [w505 w521] -> w500
                  tunnel: [w505 w510] -> w499
                  tunnel: w494 -> [_ w520]
                  tunnel: w496 -> [_ w517]
                  tunnel: w493 -> [_ w515]
                  tunnel: w492 -> [w504 w513]
                  tunnel: [w504 w513] -> w491
                  tunnel: w490 -> [w503 w512]
                  tunnel: [w502 w512] -> w489
                  tunnel: w488 -> [w501 w507]
                  tunnel: [w501 w508] -> w487
                  frame False {
                    w505 = nan
                    n212 = Increment(x=w503) -> (x+1=w502:i32)
                  }
                  frame True {
                    n213 = global read "PWAtasksGLOBAL.vi" "Probe Rotated Thro' 180"() -> (w506:bool)
                    n214 = To Double Precision Float(number=w520) -> (double precision float=w516:dbl)
                    n215 = Add(x=w520, y=i16 4095) -> (x+y=w518:i16)
                    n216 = Multiply(x=w515, y=w516) -> (x*y=w514:dbl)
                    n217 = Index Array(array=w517, index=w518) -> (element=w511:dbl)
                    n218 = Reciprocal(x=w514) -> (1/x=w521:dbl)
                    n219 = case shown="True" w506 {
                      tunnel: w511 -> [w525 w527]
                      tunnel: [w525 w526] -> w510
                      frame False {
                      }
                      frame True {
                        n220 = Negate(x=w527) -> (-x=w526:dbl)
                      }
                    }
                    n221 = Less Than 0?(x=w510) -> (x < 0?=w509:bool)
                    n222 = case shown="True" w509 {
                      tunnel: [w522 w524] -> w508
                      tunnel: w507 -> [w522 w523]
                      frame False {
                      }
                      frame True {
                        n223 = Increment(x=w523) -> (x+1=w524:i32)
                      }
                    }
                  }
                }
              }
              frame 4095 {
                w532 = 0.0 ("Eng Values")
                n224 = Increment(x=w531) -> (x+1=w530:i32)
              }
              frame -4095 {
                w537 = 0.0 ("Eng Values")
                n225 = Increment(x=w536) -> (x+1=w535:i32)
              }
            }
          }
          n226 = Build Array(w463) -> (w462:dbl[][])
          n227 = Build Array(w464) -> (w461:dbl[][])
        }
      }
      n228 = global write "PWAtasksGLOBAL.vi" "PWA 1/TOF"(w447) -> ()
      n229 = global write "PWAtasksGLOBAL.vi" "PWA No of Reverse samples"(w442) -> ()
      n230 = global write "PWAtasksGLOBAL.vi" "PWA No of  TOF Below Min"(w444) -> ()
      n231 = global write "PWAtasksGLOBAL.vi" "PWA No of  TOF Timeouts"(w443) -> ()
      n232 = global write "PWAtasksGLOBAL.vi" "PWA Data"(w446) -> ()
    }
    frame #7 {
      n233 = while {
        shift-right: [w540] -> _
        shift-left: _ -> [w538]
        stop <- FALSE continue-if-true
        n234 = call "Cluster_Analysis.vi"("Shift In"=w538) -> ("Shift Out"=w540:T12[])  [unwired: 2 in]
      }
    }
    frame #8 {
      n235 = global read "Meas_global.vi" "Analysis Info cluster"() -> (w541:T10[])
      n236 = Index Array(array=w541, index=0) -> (element=w550:T10)
      n237 = for {
        tunnel: w541 -> [w578] mode=indexing
        tunnel: [w577] -> w547 mode=indexing
        tunnel: [w565] -> w542 mode=indexing
        n238 = Unbundle By Name(w578) -> ("Total Meas Time (s)"=w565:dbl, "Inst name"=w569:string, "U"=w563:dbl, "u^2"=w572:dbl, "% u'/U"=w575:dbl, "Sd Error in Mean"=w564:dbl, "Full Stats"=w568:bool)
        n239 = call "Number_2_string.vi"("number"=w563) -> ("String"=w570:string)  [unwired: 1 in]
        n240 = call "Number_2_string.vi"("number"=w572) -> ("String"=w571:string)  [unwired: 1 in]
        n241 = Number To Fractional String(number=w575, precision (6)=i16 2) -> (F-format string=w574:string)  [unwired: 2 out]
        n242 = case shown="True" w568 {
          tunnel: [w579 w587] -> w567
          tunnel: [w579 w585] -> w566
          tunnel: w564 -> [_ w582]
          tunnel: w563 -> [_ w581]
          frame False {
            w579 = ""
          }
          frame True {
            n243 = Divide(x=w582, y=w581) -> (x/y=w583:dbl)
            n244 = Multiply(x=w583, y=100.0) -> (x*y=w580:dbl)
            n245 = call "Number_2_string.vi"("number"=w582) -> ("String"=w587:string)  [unwired: 1 in]
            n246 = Number To Fractional String(number=w580, precision (6)=i16 2) -> (F-format string=w585:string)  [unwired: 2 out]
          }
        }
        n247 = Build Array(w569, w570, w571, w574, w567, w566) -> (w573:string[])
        n248 = for {
          tunnel: [w591] -> w577 mode=indexing
          tunnel: w573 -> [w588] mode=indexing
          n249 = Equal?(x="NaN", y=w588) -> (x = y?=w592:bool)
          n250 = Select(t="", s=w592, f=w588) -> (s? t:f=w591:string)
        }
      }
      n251 = Unbundle By Name(w550) -> ("Symbol"=w552:string, "Inst type"=w551:T4)
      n252 = case shown="\"Generic Linear\"" w551 {
        tunnel: ["U" "P" "V" "tau" w597 "C" ("Symbol") "T" ("Symbol") "T" ("Symbol")] -> w549
        tunnel: w552 -> [_ _ _ _ w597 _ _ _]
        frame "Propeller anemometer", Default {
        }
        frame "Pressure Transducer" {
        }
        frame "Raw voltage" {
        }
        frame "Preston tube" {
        }
        frame "Generic Linear" {
        }
        frame "Fast FID" {
        }
        frame "Thermocouple" {
        }
        frame "Cold wire" {
        }
      }
      n253 = To Lower Case(string=w549) -> (all lower case string=w557:string)
      n254 = To Upper Case(1:w549) -> (0:w559:string)
      n255 = Format Into String(format string="%% %s'/%s", w557, w559) -> (resulting string=w558:string)  [unwired: 2 in, 1 out]
      n256 = Concatenate Strings(w557, "^2") -> (w555:string)
      n257 = Build Array("Inst name", w559, w555, w558, "Sd Err in Mean", "% Sd Err") -> (w548:string[])
      n258 = Build Array (concatenate)(w548, w547) -> (w546:string[][])
      n259 = Array Max & Min(array=w542) -> (min value=w543:dbl)  [unwired: 3 out]
      n260 = Divide(x=w543, y=60.0) -> (x/y=w544:dbl)
      n261 = global write "Meas_global.vi" "Vel stat display"(w546) -> ()
      n262 = global write "Meas_global.vi" "Actual Measurement time (min)"(w544) -> ()
    }
    frame #9 {
      n263 = global read "Dynamic_call_global.ph.vi" "Per Block Plug Ins Extra"() -> (w605:string[])
      n264 = global read "Dynamic_call_global.ph.vi" "Per Block Plug Ins"() -> (w606:string[])
      n265 = Build Array (concatenate)(w606, w605) -> (w603:string[])
      n266 = call "Analyse_string_array.vi"("String array"=w603) -> ("Unique strings"=w602:string[])  [unwired: 2 out]
      n267 = Array Size(array=w602) -> (size(s)=w604:i32)
      n268 = Greater Than 0?(x=w604) -> (x > 0?=w601:bool)
      n269 = case shown="True" w601 {
        tunnel: w602 -> [_ w607]
        frame False {
        }
        frame True {
          n270 = call "Call_Block_plug_ins.vi"("Per Block Plug Ins"=w607) -> ()
        }
      }
    }
    frame #10 {
      n271 = while {
        shift-right: [w615] -> _
        shift-left: _ -> [w614]
        shift-right: [w609] -> _
        shift-left: _ -> [w608]
        stop <- TRUE stop-if-true
        n272 = global read "Meas_global.vi" "Analysis Info cluster"() -> (w616:T10[])
        n273 = global read "Meas_global.vi" "correlate"() -> (w612:i32[][])
        n274 = global read "Meas_global.vi" "Time Trace"() -> (w610:T11[])
        n275 = for {
          tunnel: w612 -> [w635] mode=indexing
          tunnel: w616 -> [w633]
          tunnel: [w631] -> w615 mode=indexing
          tunnel: w614 -> [w630]
          tunnel: [w627] -> w611 mode=indexing
          tunnel: w610 -> [w626]
          tunnel: [w618] -> w609 mode=indexing
          tunnel: w608 -> [w617]
          i -> [w620]
          w621 = 1 items=["nearest", "linear", "spline", "cubic Hermite", "Lagrange"] ("interp. method")
          n276 = Index Array(array=w630, index=w620) -> (element=w629:T13)
          n277 = Index Array(array=w617, index=w620) -> (element=w619:T12)
          n278 = Index Array(array=w635) -> (element #1=w625:i32, element #2=w624:i32)  [unwired: 2 in]
          n279 = Index Array(array=w633, index=w625) -> (element=w634:T10)
          n280 = Index Array(array=w633, index=w624) -> (element=w632:T10)
          n281 = Index Array(array=w626, index=w625) -> (element=w623:T11)
          n282 = Index Array(array=w626, index=w624) -> (element=w622:T11)
          n283 = call "Weighted_Cross_Moments.vi"("AI Cluster 1"=w634, "AI Cluster 2"=w632, "Time Cluster 1"=w623, "Time Cluster 2"=w622, "Shift Cluster In"=w629, "Shift Input"=w619, "interp. method"=w621) -> ("Shift Output"=w618:T12, "output cluster"=w628:T14, "Shift Cluster Out"=w631:T13)  [unwired: 10 in]
          n284 = Bundle By Name(cluster=w628, "Index U"=w625, "Index W"=w624) -> (w627:T14)
        }
        n285 = global write "Meas_global.vi" "Correlation Results"(w611) -> ()
      }
    }
    frame #11 {
      n286 = global read "Meas_global.vi" "Correlation Results"() -> (w640:T14[])
      n287 = global read "Meas_global.vi" "Vel stat display"() -> (w637:string[][])
      n288 = Array Size(array=w640) -> (size(s)=w639:i32)
      n289 = Greater Than 0?(x=w639) -> (x > 0?=w638:bool)
      n290 = case shown="True" w638 {
        tunnel: w640 -> [_ w650]
        tunnel: w637 -> [w641 w643]
        tunnel: [w641 w642] -> w636
        frame False {
        }
        frame True {
          n291 = for {
            tunnel: [w657] -> w645 mode=indexing
            tunnel: w650 -> [w656] mode=indexing
            n292 = Unbundle By Name(w656) -> ("U inst"=w659:string, "W inst"=w658:string, "uw"=w652:dbl, "uw/u'w'"=w654:dbl)
            n293 = call "Number_2_string.vi"("number"=w652) -> ("String"=w651:string)  [unwired: 1 in]
            n294 = Number To Fractional String(number=w654, precision (6)=i16 3) -> (F-format string=w653:string)  [unwired: 2 out]
            n295 = Build Array(w659, w658, w651, w653) -> (w657:string[])
          }
          n296 = Build Array("u inst", "w inst", "uw", "uw/u'w'") -> (w644:string[])
          n297 = Build Array (concatenate)(w643, w644, w645) -> (w642:string[][])
        }
      }
      "Vel stat display" <- w636
      n298 = global write "Meas_global.vi" "Vel stat display"(w636) -> ()
    }
    frame #12 {
      n299 = call "Voltage_overflow_checker.vi"("Voltages"=w660) -> ()  [unwired: 3 out]
    }
    frame #13 {
      # "And declare \"Time's up\" if the error is good enough"
      # "..and the multirun row has valid skip settings in its Extra Commands fiield, and the skip channel has measured long enough to meet its minimum time..."
      # "If we're in a live multirun..."
      n300 = global read "Meas_global.vi" "Post Process"() -> (w665:T5)
      n301 = Equal?(x=w665, y=Post_Process."Take New Data" ("Post Process")) -> (x = y?=w664:bool)
      n302 = global read "Meas_global.vi" "Analysis Info cluster"() -> (w661:T10[])
      n303 = Compound Arithmetic op=AND(w664, invert "Measurement top level?") -> (w662:bool)
      n304 = case shown="True" w662 {
        tunnel: ["" ("Instrument Code Name") w676] -> w670
        tunnel: [0.0 ("Sd Error Theshold value") w675] -> w669
        tunnel: [FALSE w674] -> w667
        frame False {
        }
        frame True {
          n305 = global read "Trav_pos_global.vi" "Current Row"() -> (w677:T15)
          n306 = global read "Meas_global.vi" "Actual Measurement time (min)"() -> (w684:dbl)
          n307 = Unbundle By Name(w677) -> ("Extra Commands"=w678:string)
          n308 = call "Skip_If Sd_Error_Below.vi"("String to Search"=w678, "Simulate/Run"=User_Specific_mode."Run VI", "Measurement setup Applied?"=FALSE) -> ("Check for Skip?"=w682:bool, "Instrument Code Name"=w676:string, "Sd Error Theshold value"=w675:dbl, "Minimum Measurement time (Sec)"=w681:dbl)  [unwired: 2 in, 1 out]
          n309 = Multiply(x=w684, y=60.0) -> (x*y=w686:dbl)
          n310 = Greater Or Equal?(x=w686, y=w681) -> (x >= y?=w683:bool)
          n311 = Compound Arithmetic op=AND(w682, w683) -> (w674:bool)
        }
      }
      n312 = case shown="True" w667 {
        tunnel: w670 -> [_ w691]
        tunnel: w669 -> [_ w690]
        tunnel: [FALSE w689] -> w668
        tunnel: w661 -> [_ w688]
        frame False {
        }
        frame True {
          # "...then check the standard error against the skip threshold"
          n313 = for {
            tunnel: w688 -> [w695] mode=indexing
            tunnel: [w694] -> w692 mode=indexing
            n314 = Unbundle By Name(w695) -> ("Code name"=w697:string)
            n315 = Match Pattern(string=w697, regular expression=":") -> (before substring=w694:string)  [unwired: 4 out]
          }
          n316 = Search 1D Array(1D array=w692, element=w691) -> (index of element=w693:i32)  [unwired: 1 out]
          n317 = case shown="0, Default" w693 {
            tunnel: w693 -> [w703 _]
            tunnel: [w701 FALSE] -> w689
            tunnel: w690 -> [w700 _]
            tunnel: w688 -> [w699 _]
            frame 0, Default {
              n318 = Index Array(array=w699, index=w703) -> (element=w702:T10)
              n319 = Unbundle By Name(w702) -> ("Sd Error in Mean"=w698:dbl)
              n320 = Less?(x=w698, y=w700) -> (x < y?=w701:bool)
            }
            frame -1 {
            }
          }
        }
      }
      "Max Measurement time up" <- w668
    }
    frame #14 {
      n321 = global read "Meas_global.vi" "Second Graph"() -> (w707:T19)
      n322 = global read "Meas_global.vi" "First Graph"() -> (w705:T19)
      n323 = call "Create_Plot.vi"("First Graph"=w705) -> ("Array"=→"First Plot data Cluster":cluster{"X array":dbl[], "Y array":dbl[]}[])
      n324 = call "Create_Plot.vi"("First Graph"=w707) -> ("Array"=→"Second Plot Data Cluster":cluster{"X array":dbl[], "Y array":dbl[]}[])
    }
    frame #15 {
      n325 = case shown="\"Take LDA data\"" w710 {
        tunnel: [FALSE w712] -> w709
        frame "No LDA data" {
        }
        frame "Take LDA data" {
          n326 = global read "Meas_global.vi" "Analysis Info cluster"() -> (w715:T10[])
          n327 = global read "Preference_global.vi" "Server Comms"() -> (w719:T8)
          n328 = global read "Meas_global.vi" "Post Process"() -> (w716:T5)
          n329 = global read "Meas_global.vi" "File"() -> (w722:T7)
          n330 = Equal?(x=w722, y=T7."Save no data" ("File")) -> (x = y?=w724:bool)
          n331 = for {
            tunnel: w715 -> [w734] mode=indexing
            tunnel: [w728] -> w714 mode=indexing if=w729
            n332 = Unbundle By Name(w734) -> ("Av Sampling Rate"=w728:dbl, "Inst type"=w732:T4)
            n333 = Not A Number/Path/Refnum?(number/path/refnum=w728) -> (NaN/Path/Refnum?=w730:bool)
            n334 = Absolute Value(x=w728) -> (abs(x)=w727:dbl)
            n335 = Equal?(x=w732, y=Inst_type."LDA Vel" ("Inst type")) -> (x = y?=w731:bool)
            n336 = Not Equal?(x=w727, y=inf) -> (x != y?=w725:bool)
            n337 = Compound Arithmetic op=AND(w725, invert w730, w731) -> (w729:bool)
          }
          n338 = Equal?(x=w716, y=Post_Process."Take New Data" ("Post Process")) -> (x = y?=w721:bool)
          n339 = Equal?(x=w719, y=Server_Comms."Server Link Healthy" ("Server Comms")) -> (x = y?=w720:bool)
          n340 = Compound Arithmetic op=AND(invert w724, w721, w720) -> (w712:bool)
          n341 = Array Max & Min(array=w714) -> (min value=w713:dbl)  [unwired: 3 out]
          n342 = global write "Meas_global.vi" "Actual Sampling rate (Hz)"(w713) -> ()
        }
      }
    }
    frame #16 {
      n343 = case shown="True" w735 {
        frame False {
        }
        frame True {
          w737 = 2.0 ("y")
          n344 = global read "Meas_global.vi" "Actual Sampling rate (Hz)"() -> (w738:dbl)
          n345 = global read "Preference_global.vi" "Rig Setup"() -> (w740:string)
          n346 = Greater?(x=w738, y=w737) -> (0:w739:bool)
          n347 = Select(t=w738, s=w739, f=w737) -> (s? t:f=w736:dbl)
          n348 = while {
            shift-right: [w749] -> _
            shift-left: _ -> [w743]
            shift-right: [w745] -> _
            shift-left: _ -> [w748]
            tunnel: w740 -> [w742]
            tunnel: w736 -> [w741]
            stop <- TRUE stop-if-true
            n349 = global read "Meas_global.vi" "Requested Sampling rate"() -> (w746:dbl)
            n350 = Get Date/Time In Seconds() -> (seconds since 1Jan1904=w751:timestamp)
            n351 = To Double Precision Float(number=w751) -> (double precision float=w744:dbl)
            n352 = Build Array (concatenate)(w748, w741) -> (w747:dbl[])
            n353 = case shown="\"Enflo_Tunnel\", Default" w742 {
              tunnel: [w762 w785] -> w749
              tunnel: w744 -> [w761 w785]
              tunnel: w747 -> [w760 w786]
              tunnel: w746 -> [w759 w784]
              tunnel: [w758 w786] -> w745
              tunnel: w741 -> [w757 w783]
              tunnel: w744 -> [w755 _]
              tunnel: w743 -> [w754 _]
              frame "Enflo_Tunnel", Default {
                n354 = Subtract(x=w755, y=w754) -> (x-y=w752:dbl)
                n355 = Greater?(x=w752, y=180.0) -> (0:w753:bool)
                n356 = case shown="True" w753 {
                  tunnel: [w764 w777] -> w762
                  tunnel: w761 -> [_ w777]
                  tunnel: w754 -> [w764 _]
                  tunnel: w760 -> [w763 w769]
                  tunnel: w759 -> [_ w773]
                  tunnel: w757 -> [_ w766]
                  tunnel: [w763 dbl[] []] -> w758
                  tunnel: w752 -> [_ w771]
                  frame False {
                  }
                  frame True {
                    w775 = 10.0  # In range %
                    n357 = call "Mean_fr_NaN_data.vi"("Data"=w769) -> ("Mean value"=w767:dbl)  [unwired: 1 out]
                    n358 = Less?(x=w771, y=60.0) -> (x < y?=w768:bool)
                    n359 = Select(t=w767, s=w768, f=w766) -> (s? t:f=w765:dbl)
                    n360 = call "Hydrosonic_Conrol.vi"("In range %"=w775, "Input Mode"=enum16{"Desired Frequency", "Transducer value"}."Desired Frequency", "Actual Sampling rate (Hz)"=w765, "Desired Value"=w773) -> ("Set output"=w774:dbl)  [unwired: 1 out]
                    n361 = call "Display_LDA_data_rate.vi"("Hydrosonic Setting %"=w774, "Current Sampling Freq (Hz)"=w766) -> ()  [unwired: 1 out]
                  }
                }
              }
              frame "Aero_Tunnel" {
                n362 = Build Array("Aero_Tunnel:Motor:Enable" ("Channel Name")) -> (w782:string[])
                n363 = call "Get_Current_Scan_client.vi"("ADAM Ch Names"=w782) -> ("Numerical Values"=w780:dbl[])  [unwired: 3 out]
                n364 = Index Array(array=w780) -> (element=w779:dbl)  [unwired: 1 in]
                n365 = Equal To 0?(x=w779) -> (x = 0?=w778:bool)
                n366 = case shown="False" w778 {
                  tunnel: w784 -> [w794 _]
                  tunnel: w783 -> [w791 w798]
                  frame False {
                    n367 = Multiply(x=1.05, y=w794) -> (x*y=w793:dbl)
                    n368 = Greater Or Equal?(x=w791, y=w793) -> (x >= y?=w797:bool)
                    n369 = Select(t=0.0, s=w797, f=1.0) -> (s? t:f=w788:dbl)
                    n370 = call "Display_LDA_data_rate.vi"("Hydrosonic Setting %"=w788, "Current Sampling Freq (Hz)"=w791) -> ()  [unwired: 1 out]
                    n371 = Build Array("Aero_Tunnel:Seeder:Enable" ("Channel Name")) -> (w789:string[])
                    n372 = Build Array(w788) -> (w787:dbl[])
                    n373 = call "ASYNC_Adam_client.vi"("Values"=w787, "Channel Names"=w789) -> ()  [unwired: 1 in, 2 out]
                  }
                  frame True {
                    # "Control Seeder Manually"
                    n374 = call "Display_LDA_data_rate.vi"("Current Sampling Freq (Hz)"=w798) -> ()  [unwired: 1 in, 1 out]
                  }
                }
              }
            }
          }
        }
      }
    }
  }
